vi "CreateSignal.vi"(7 "dt":dbl, 9 "t0_1":dbl, 10 "PronyEstimate":dbl[](array[numeric]), 11 "InputSignal":dbl[](array[numeric])) -> (0 "DynamicPronyEstimate":dynamicdata(graph), 2 "DynamicInputSignal":dynamicdata(graph))   [LabVIEW 2017, in "Visualization.lvlib" / "VisualizeAppRingdown.lvclass"]
uses:
  VisualizeAppRingdown.lvclass
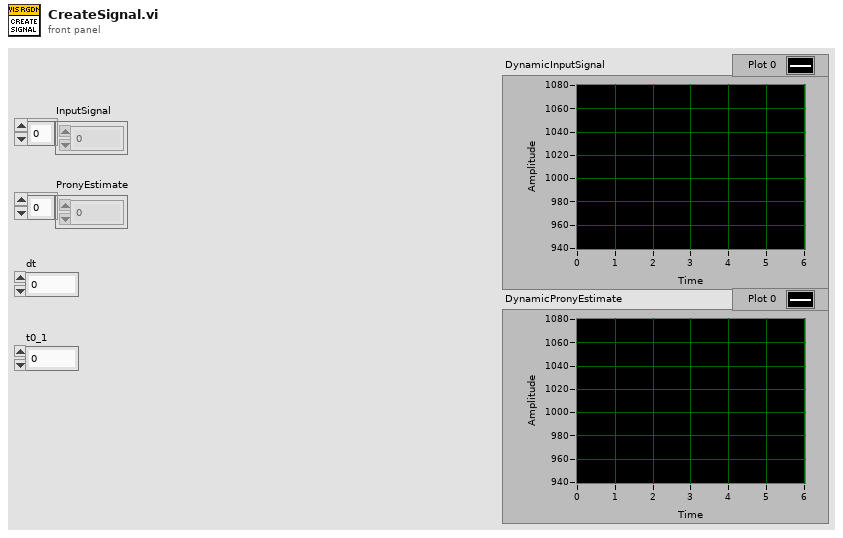
[diagram p1: front panel]
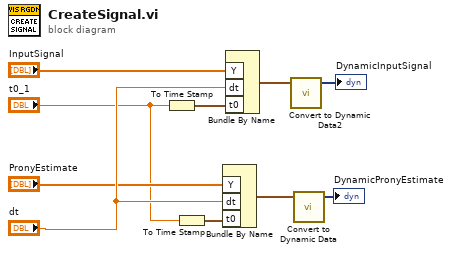
[diagram p0: block diagram]
diagram:
  n1 = To Time Stamp(1:"t0_1") -> (0:w7:timestamp)
  n2 = To Time Stamp(1:"t0_1") -> (0:w6:timestamp)
  n3 = Bundle By Name("Y"="PronyEstimate", "dt"="dt", "t0"=w6) -> (w4:waveform(dbl))  [unwired: 1 in]
  n4 = Bundle By Name("Y"="InputSignal", "dt"="dt", "t0"=w7) -> (w5:waveform(dbl))  [unwired: 1 in]
  n5 = call "Convert to Dynamic Data2"("Waveform"=w5) -> ("Dynamic Data Type"=→"DynamicInputSignal":dynamicdata)  [unwired: 3 in]
  n6 = call "Convert to Dynamic Data"("Waveform"=w4) -> ("Dynamic Data Type"=→"DynamicPronyEstimate":dynamicdata)  [unwired: 3 in]
